vi "LMS_Init.vi"(8 "error in (no error)":errorcluster, 11 "device_In":i64) -> (0 "error out":errorcluster, 3 "device_Out":i64)   [LabVIEW 2018, in "LMS_LV_Drv.lvlib"]
uses:
  LMS_LV_Drv.lvlib
  C:/Program Files/PothosSDR/bin/LimeSuite.dll
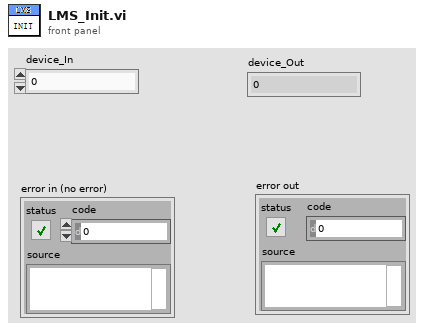
[diagram p1: front panel]
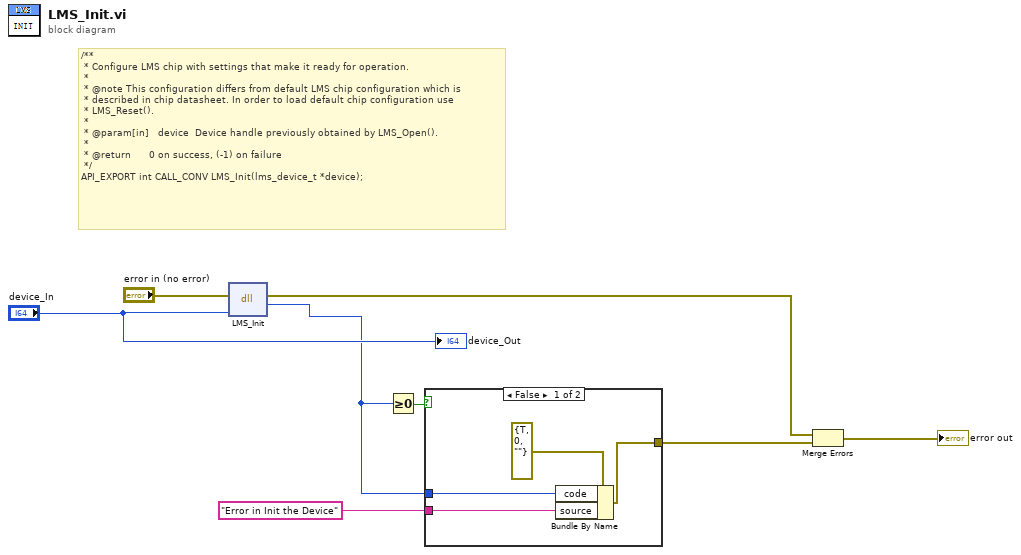
[diagram p0: block diagram]
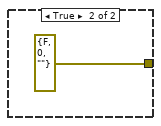
[diagram p2: hidden frame]
diagram:
  # "/**\n * Configure LMS chip with settings that make it ready for operation.\n *\n * @note This configuration differs from default LMS chip configuration which is\n * described in chip datasheet. In order to load default chip configuration use\n * LMS_Reset().\n *\n * @param[in]   device  Device handle previously obtained by LMS_Open().\n *\n * @return      0 on success, (-1) on failure\n */\nAPI_EXPORT int CALL_CONV LMS_Init(lms_device_t *device);"
  n1 = dll-call lib="C:/Program Files/PothosSDR/bin/LimeSuite.dll" fn="LMS_Init"(error in="error in (no error)", "device"="device_In") -> (error out=w3:errorcluster, "return type"=w4:i32)  [unwired: 3 in, 1 out]
  n2 = Greater Or Equal To 0?(x=w4) -> (x >= 0?=w6:bool)
  n3 = case shown="False" w6 {
    tunnel: [w11 errorcluster {"status"=FALSE, "code"=0, "source"=""} ("error in")] -> w1
    tunnel: w4 -> [w10 _]
    tunnel: "Error in Init the Device" ("source") -> [w9 _]
    frame False {
      n4 = Bundle By Name(cluster=errorcluster {"status"=TRUE, "code"=0, "source"=""} ("error in"), "code"=w10, "source"=w9) -> (w11:errorcluster)
    }
    frame True {
    }
  }
  n5 = Merge Errors(w3, w1) -> (→"error out":errorcluster)
  "device_Out" <- "device_In"
